vi "RDS Serial Read Config.vi"(8 "error in (no error)":errorcluster, 11 "RDS Serial Instrument Actor in":refnum<class "RDS Serial Instrument Actor.lvclass">) -> (0 "error out":errorcluster, 1 "baud rate (9600)":u32, 2 "VISA resource name":refnum<visa-resource-name>, 3 "RDS Serial Instrument Actor out":refnum<class "RDS Serial Instrument Actor.lvclass">, 5 "Termination Char(s)":string)   [LabVIEW 2015, in "RDS Abstracts.lvlib" / "RDS Serial Instrument Actor.lvlib" / "RDS Serial Instrument Actor.lvclass"]
uses:
  RDS Serial Instrument Actor.lvclass
  RDS Serial Instrument Actor.lvclass/RDS Serial Instrument Actor.ctl
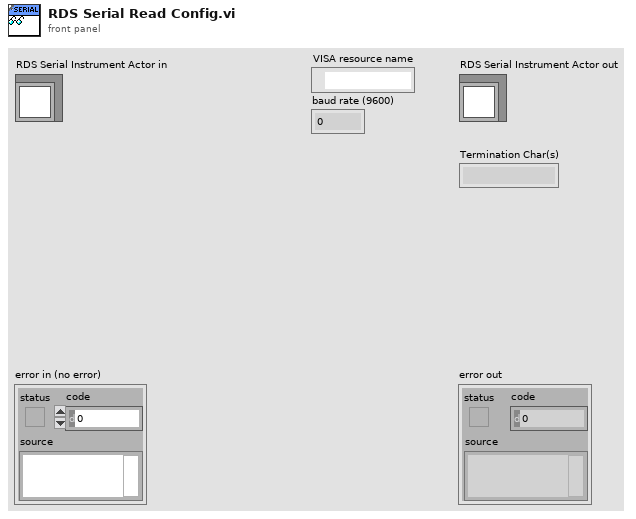
[diagram p1: front panel]
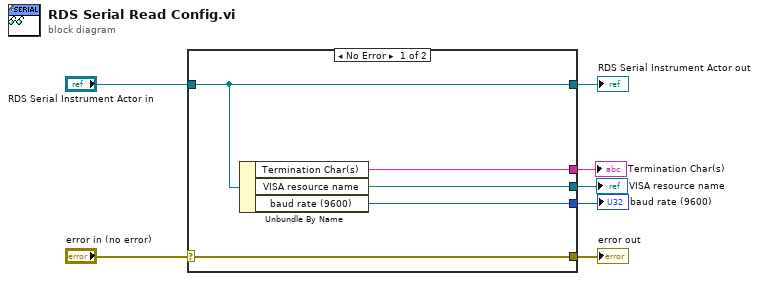
[diagram p0: block diagram]
diagram:
  n1 = case shown="No Error" "error in (no error)" {
    selector: "error in (no error)" -> [w12 w13]
    tunnel: [w12 w13] -> w6
    tunnel: [w11 w14] -> w4
    tunnel: "RDS Serial Instrument Actor in" -> [w11 w14]
    tunnel: [w10 _] -> w3
    tunnel: [w9 _] -> w2
    tunnel: [w8 _] -> w1
    frame No Error {
      n2 = Unbundle By Name(w11) -> ("Termination Char(s)"=w10:string, "VISA resource name"=w9:refnum<visa-resource-name>, "baud rate (9600)"=w8:u32)
    }
    frame Error {
    }
  }
  "error out" <- w6
  "RDS Serial Instrument Actor out" <- w4
  "Termination Char(s)" <- w3
  "VISA resource name" <- w2
  "baud rate (9600)" <- w1
